vi "Configure FM Internal [FM] Core.vi"(7 "modulation waveform (Sine)":i32(ring)=1 items=["Sine"=1, "Square"=2, "Triangle"=3, "Ramp Up"=4, "Ramp Down"=5], 8 "error in (no error)":errorcluster, 9 "modulation frequency (1000 Hz)":dbl[unit]=1000.0 format="%^.2e", 10 "peak deviation (100 Hz)":dbl[unit]=100.0 format="%^.2e", 11 "CS++Fgen in":refnum<class "CS++Fgen.lvclass">) -> (0 "error out":errorcluster, 3 "CS++Fgen out":refnum<class "CS++Fgen.lvclass">)   [LabVIEW 2016, in "CS++Fgen.lvlib" / "CS++Fgen.lvclass"]
doc: "This VI configures the properties that control the function generator's internal frequency modulation source. These properties are the peak deviation, waveform, and frequency.\n\nNotes:\n\n(1) This VI is part of the IviFgenModulateFM [FM] extension group."
uses:
  CS++Fgen.lvclass
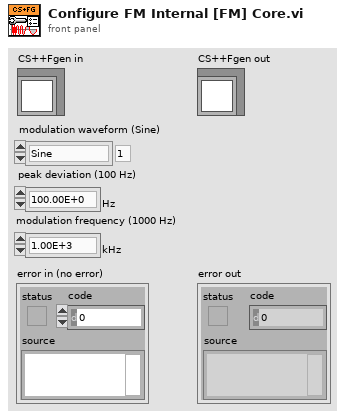
[diagram p1: front panel]
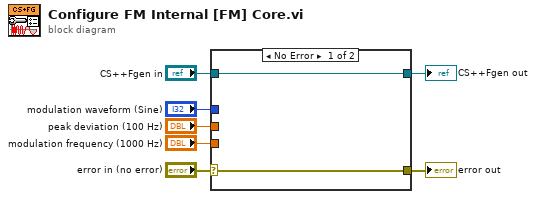
[diagram p0: block diagram]
diagram:
  n1 = case shown="No Error" "error in (no error)" {
    selector: "error in (no error)" -> [w8 w11]
    tunnel: [w8 w11] -> w6
    tunnel: [w9 w10] -> w4
    tunnel: "CS++Fgen in" -> [w9 w10]
    tunnel: "modulation waveform (Sine)" -> [_ _]
    tunnel: "peak deviation (100 Hz)" -> [_ _]
    tunnel: "modulation frequency (1000 Hz)" -> [_ _]
    frame No Error {
    }
    frame Error {
    }
  }
  "error out" <- w6
  "CS++Fgen out" <- w4
